vi "DeCoF remote command.vi"(6 "error in (no error)":errorcluster, 7 "time out (ms)":i32=2000, 8 "command":string, 9 "Conncection ID in":T1) -> (0 "error out":errorcluster, 1 "timed out?":bool, 2 "answer string":string, 3 "Conncection ID out":T1, 4 "complete answer":string)   [LabVIEW 2013]
doc: "This VI sends a command string to the remote device, waits until it returns an answer or a timeout expires.\nIf the answer contains \"ERROR\" the error out cluster returns error 9999."
uses:
  subVIs/DeCoF connection.ctl
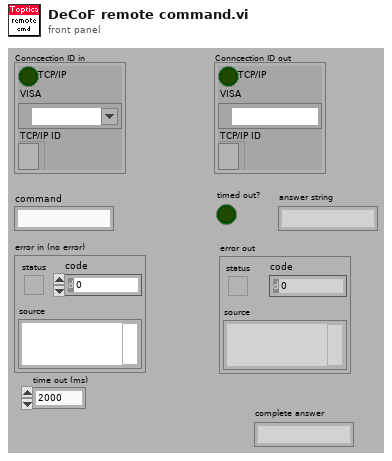
[diagram p1: front panel]
types:
  T1 = typedef "DeCoF connection.ctl" = cluster{"TCP/IP":bool, "VISA":refnum<visa-resource-name>, "TCP/IP ID":refnum<k5>}
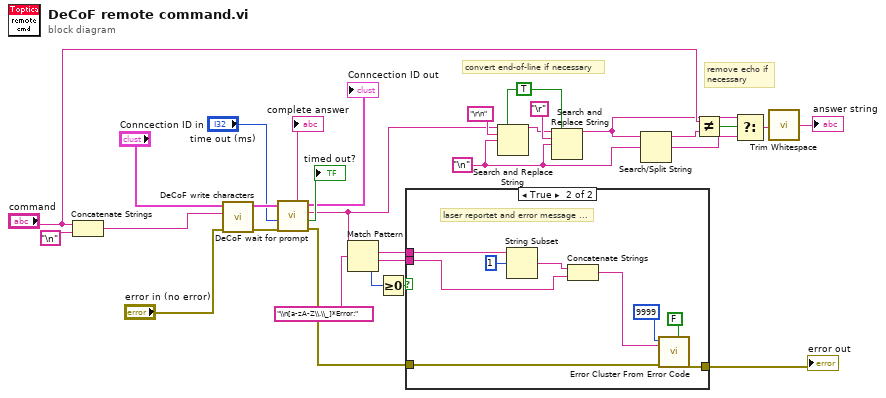
[diagram p0: block diagram]
diagram:
  w13 = TRUE ("replace all? (F)")
  w8 = "\n" ("search string")
  # "remove echo if\nnecessary"
  # "convert end-of-line if necessary"
  n1 = Concatenate Strings("command", "\n") -> (w9:string)
  n2 = call "DeCoF write characters.vi"("error in (no error)"="error in (no error)", "data in"=w9, "Connection ID in"="Conncection ID in") -> ("error out"=w30:errorcluster, "Conncection ID out"=w29:T1)  [unwired: 3 in]
  n3 = call "DeCoF wait for prompt.vi"("Connection ID in"=w29, "time out (ms)"="time out (ms)", "error in (no error)"=w30) -> ("complete answer"=→"complete answer":string, "Conncection ID out"=→"Conncection ID out":T1, "answer string"=w10:string, "timed out?"=→"timed out?":bool, "error out"=w24:errorcluster)  [unwired: 1 in]
  n4 = Match Pattern(string=w10, regular expression="\\n[a-zA-Z\\.\\_]*Error:") -> (match substring=w17:string, after substring=w15:string, offset past match=w16:i32)  [unwired: 1 in, 1 out]
  n5 = Greater Or Equal To 0?(x=w16) -> (x >= 0?=w25:bool)
  n6 = case shown="True" w25 {
    tunnel: [w31 w40] -> w23
    tunnel: w24 -> [w31 w38]
    tunnel: w17 -> [_ w36]
    tunnel: w15 -> [_ w33]
    frame False {
    }
    frame True {
      # "laser reportet and error message ..."
      n7 = String Subset(string=w36, offset (0)=1) -> (substring=w34:string)  [unwired: 1 in]
      n8 = Concatenate Strings(w34, w33) -> (w32:string)
      n9 = call <vilib>:"Error Cluster From Error Code.vi"("is warning? (False)"=FALSE, "error in (no error)"=w38, "error message (\"\")"=w32, "error code (0)"=9999) -> ("error out"=w40:errorcluster)  [unwired: 5 in]
    }
  }
  "error out" <- w23
  n10 = Search and Replace String(replace all?=w13, input string=w10, search string="\r\n", replace string=w8) -> (result string=w11:string)  [unwired: 4 in, 3 out]
  n11 = Search and Replace String(replace all?=w13, input string=w11, search string="\r", replace string=w8) -> (result string=w4:string)  [unwired: 4 in, 3 out]
  n12 = Search/Split String(string=w4, search string/char (-)=w8) -> (substring before match=w7:string, match + rest of string=w3:string)  [unwired: 1 in, 1 out]
  n13 = Not Equal?(x="command", y=w7) -> (x != y?=w5:bool)
  n14 = Select(t=w4, s=w5, f=w3) -> (s? t:f=w2:string)
  n15 = call <vilib>:"Trim Whitespace.vi"("string"=w2) -> ("trimmed string"=→"answer string":string)  [unwired: 1 in]
